vi "transmitter_labview.vi"() -> ()   [LabVIEW 2025]
uses:
  <vilib>/Instr/_visa.llb/VISA Configure Serial Port (Instr).vi
panel:
  in  "timeout (10sec)":u32=10000
  out "output string":string
  out "Raw string":string
  in  "Reverse":bool
  in  "Forward":bool
  out "Temperature":string
  out "Motor Speed (RPM)":string
  out "LDR Level":string
  out "Humidity":string
  out "Motor feedback":dbl(graph)
  in  "Start PID":bool
  in  "Motor Speed (RPM) / PWM (Manual)":u16 max=100 step=5
  in  "stop bits (10: 1 bit)":u16(ring)=10 items=["1.0"=10, "1.5"=15, "2.0"=20]
  in  "parity (0:none)":enum16{"None", "Odd", "Even", "Mark", "Space"}(ring)
  in  "data bits (8)":u16=8 min=5 max=8 step=1
  in  "baud rate (9600)":u32=9600
  in  "?":bool
  in  "Stop":bool
  in  "VISA resource COM PORT":refnum<visa-resource-name>
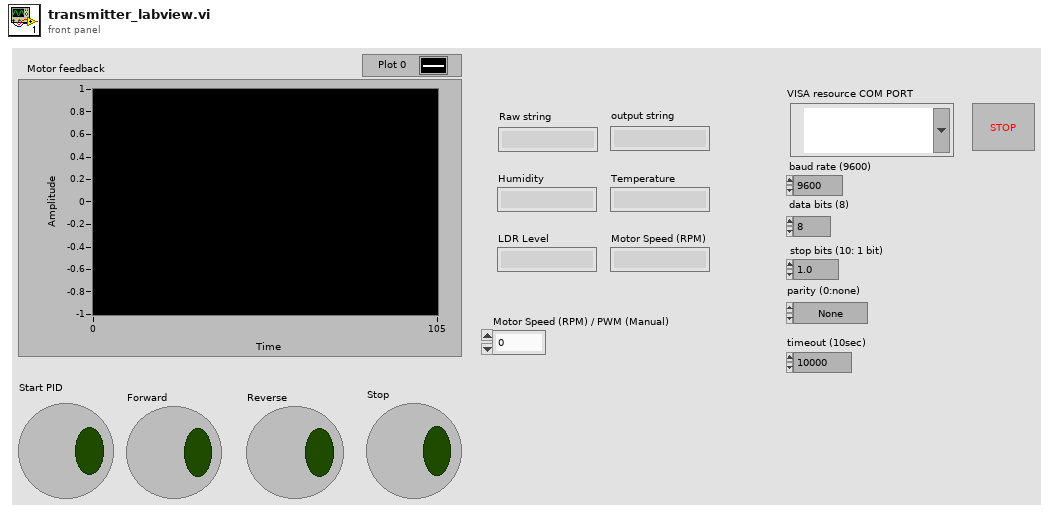
[diagram p1: front panel]
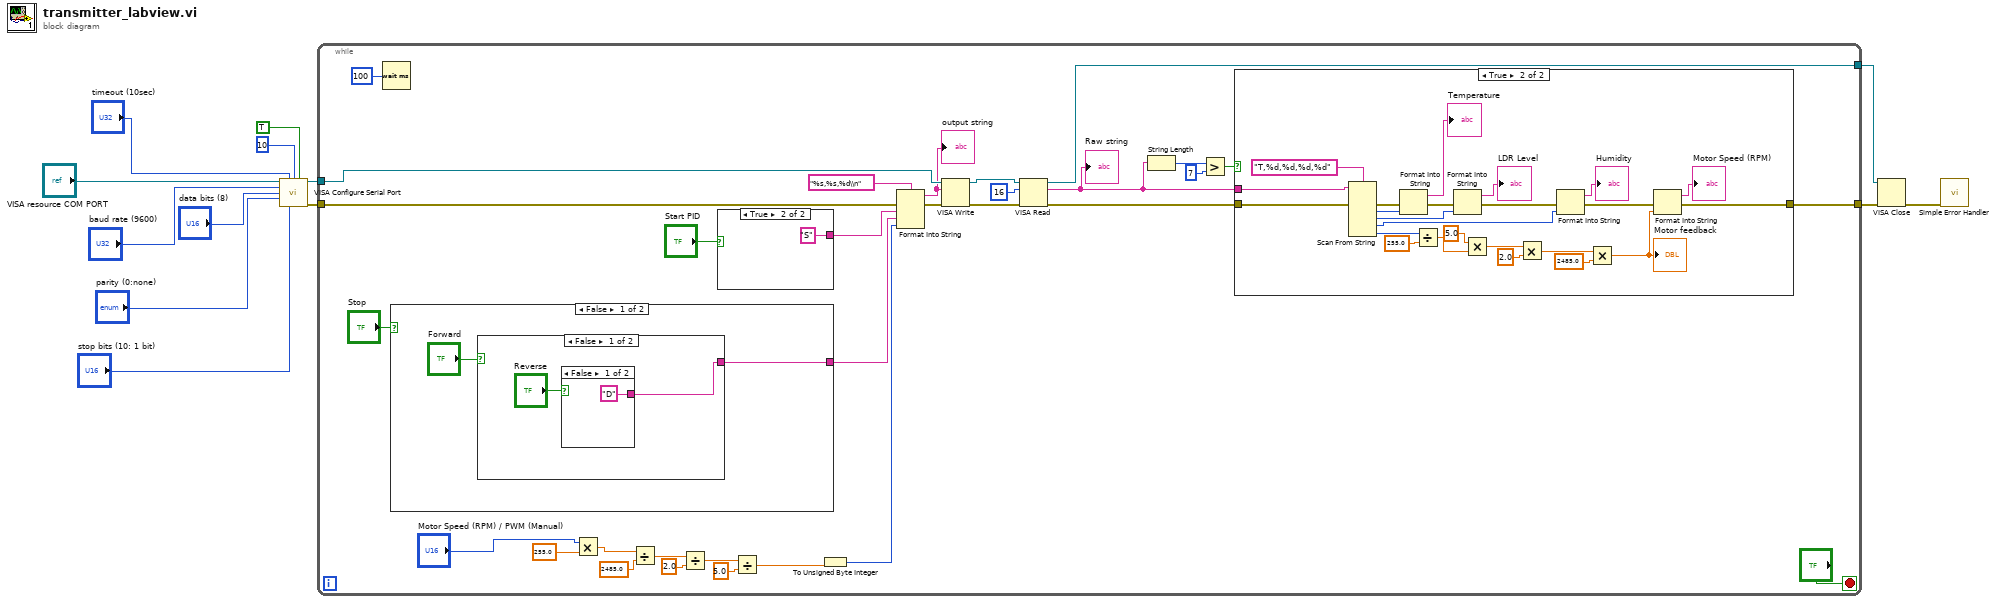
[diagram p0: block diagram]
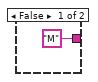
[diagram p3: hidden frame]
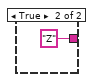
[diagram p4: hidden frame]
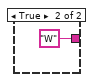
[diagram p5: hidden frame]
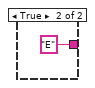
[diagram p6: hidden frame]
diagram:
  n1 = call-poly "VISA Configure Serial Port"("VISA resource name"="VISA resource COM PORT", "timeout (10sec)"="timeout (10sec)", "termination char\n(0xA = '\\n' = LF)"=u8 10 ("termination char\n(0xA = '\\n' = LF)"), "Enable Termination\nChar (T)"=TRUE ("Enable Termination\nChar (T)"), "baud rate (9600)"="baud rate (9600)", "data bits (8)"="data bits (8)", "parity (0:none)"="parity (0:none)", "stop bits (10: 1 bit)"="stop bits (10: 1 bit)") -> ("VISA resource name out"=w7:refnum<visa-resource-name>, "error out"=w6:errorcluster)  [unwired: 6 in]
  n2 = while {
    tunnel: w6 -> [w28]
    tunnel: w7 -> [w33]
    tunnel: [w39] -> w4
    tunnel: [w29] -> w3
    stop <- "?" stop-if-true
    n3 = Wait (ms)(milliseconds to wait=u32 100 ("millisecond timer value")) -> ()  [unwired: 1 out]
    n4 = case shown="False" "Stop" {
      tunnel: [w72 "E" ("write buffer")] -> w34
      frame False {
        n5 = case shown="False" "Forward" {
          tunnel: [w74 "W" ("write buffer")] -> w72
          frame False {
            n6 = case shown="False" "Reverse" {
              tunnel: ["D" ("write buffer") "Z" ("write buffer")] -> w74
              frame False {
              }
              frame True {
              }
            }
          }
          frame True {
          }
        }
      }
      frame True {
      }
    }
    n7 = Multiply(x="Motor Speed (RPM) / PWM (Manual)", y=255.0) -> (x*y=w16:dbl)
    n8 = Divide(x=w16, y=2485.0) -> (x/y=w22:dbl)
    n9 = Divide(x=w22, y=2.0) -> (x/y=w20:dbl)
    n10 = case shown="True" "Start PID" {
      tunnel: ["M" ("write buffer") "S" ("write buffer")] -> w35
      frame False {
      }
      frame True {
      }
    }
    n11 = Divide(x=w20, y=5.0) -> (x/y=w15:dbl)
    n12 = To Unsigned Byte Integer(number=w15) -> (unsigned 8bit integer=w14:u8)
    n13 = Format Into String(format string="%s,%s,%d\\n", error in=w28, w35, w34, w14) -> (resulting string=w31:string, error out=w27:errorcluster)  [unwired: 1 in]
    "output string" <- w31
    n14 = VISA Write(VISA resource name=w33, write buffer=w31, error in (no error)=w27) -> (VISA resource name out=w38:refnum<visa-resource-name>, error out=w37:errorcluster)  [unwired: 1 out]
    n15 = VISA Read(VISA resource name=w38, byte count=u32 16, error in (no error)=w37) -> (VISA resource name out=w39:refnum<visa-resource-name>, read buffer=w32:string, error out=w30:errorcluster)  [unwired: 1 out]
    "Raw string" <- w32
    n16 = String Length(string=w32) -> (length=w25:i32)
    n17 = Greater?(x=w25, y=7) -> (0:w26:bool)
    n18 = case shown="True" w26 {
      tunnel: w32 -> [_ w62]
      tunnel: w30 -> [w45 w61]
      tunnel: [w45 w56] -> w29
      frame False {
      }
      frame True {
        n19 = Scan From String(format string="T,%d,%d,%d,%d", input string=w62, error in=w61) -> (error out=w60:errorcluster, output 1=w67:i32, output 2=w68:i32, output 3=w69:i32, output 4=w54:i32)  [unwired: 5 in, 2 out]
        n20 = Format Into String(error in=w60, w67) -> (resulting string=→"Temperature":string, error out=w59:errorcluster)  [unwired: 2 in]
        n21 = Divide(x=w54, y=255.0) -> (x/y=w52:dbl)
        n22 = Format Into String(error in=w59, w68) -> (resulting string=→"LDR Level":string, error out=w58:errorcluster)  [unwired: 2 in]
        n23 = Multiply(x=5.0, y=w52) -> (x*y=w50:dbl)
        n24 = Multiply(x=w50, y=2.0) -> (x*y=w48:dbl)
        n25 = Format Into String(error in=w58, w69) -> (resulting string=→"Humidity":string, error out=w57:errorcluster)  [unwired: 2 in]
        n26 = Multiply(x=w48, y=2485.0) -> (x*y=w46:dbl)
        "Motor feedback" <- w46
        n27 = Format Into String(error in=w57, w46) -> (resulting string=→"Motor Speed (RPM)":string, error out=w56:errorcluster)  [unwired: 2 in]
      }
    }
  }
  n28 = VISA Close(VISA resource name=w4, error in (no error)=w3) -> (error out=w5:errorcluster)
  n29 = call <vilib>:"Simple Error Handler.vi"("error in (no error)"=w5) -> ()  [unwired: 4 in, 5 out]
